vi "Configure DC Voltage Filter.vi"(8 "error in (no error)":errorcluster, 10 "Enable DC Voltage Filter (Disable)":bool, 11 "VISA resource name":refnum<visa-resource-name>) -> (0 "error out":errorcluster, 3 "VISA resource name out":refnum<visa-resource-name>)   [LabVIEW 2020, in "Library Instrument & Equipement.lvlib" / "Library Multimeter.lvlib" / "RIGOL DM3058.lvlib"]
doc: "Configures the DC Voltage Filter.\n\n<B>Note:</B>\nThis VI only applies to RIGOL DM3058 model."
uses:
  RIGOL DM3058.lvlib
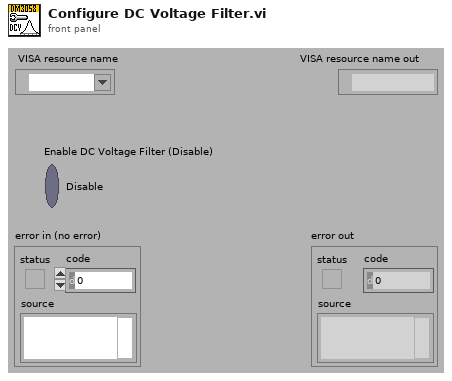
[diagram p1: front panel]
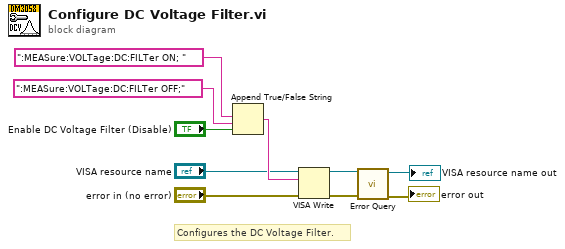
[diagram p0: block diagram]
diagram:
  # "Configures the DC Voltage Filter."
  n1 = Append True/False String(1:"Enable DC Voltage Filter (Disable)", 2:":MEASure:VOLTage:DC:FILTer OFF;", 3:":MEASure:VOLTage:DC:FILTer ON; ") -> (0:w7:string)  [unwired: 1 out]
  n2 = VISA Write(VISA resource name="VISA resource name", write buffer=w7, error in (no error)="error in (no error)") -> (VISA resource name out=w4:refnum<visa-resource-name>, error out=w3:errorcluster)  [unwired: 1 out]
  n3 = call "Error Query.vi"("error in (no error)"=w3, "VISA resource name"=w4) -> ("error out"=→"error out":errorcluster, "VISA resource name out"=→"VISA resource name out":refnum<visa-resource-name>)  [unwired: 6 in, 2 out]
